vi "XNET Read (Frame Raw).vi"(0 "session in":refnum<k21>, 7 "number to read (-1)":i32=-1, 9 "timeout (0)":dbl format="%.2g", 11 "error in (no error)":errorcluster) -> (4 "session out":refnum<k21>, 6 "data":u8[](array[numeric]) format="%02x", 15 "error out":errorcluster)   [LabVIEW 2018]
doc: "Reads data from a session as an array of raw bytes. The session must use a mode of Frame Input Stream, Frame Input Queued, or Frame Input Single-Point."
uses:
  nixlvapi.dll
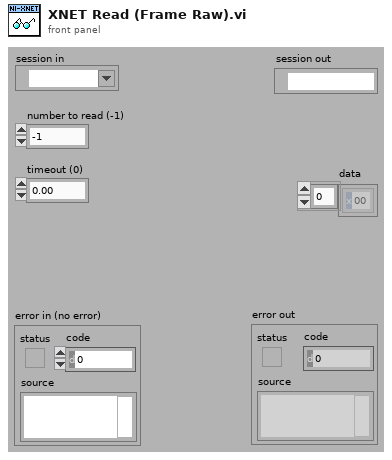
[diagram p1: front panel]
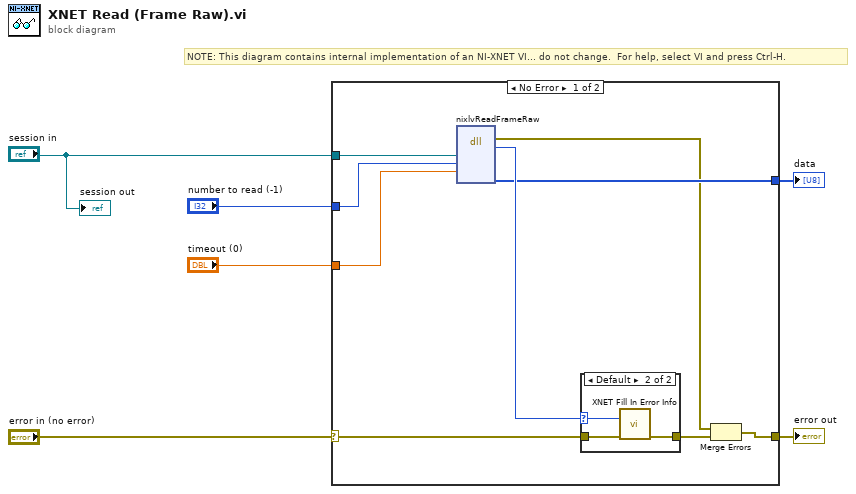
[diagram p0: block diagram]
diagram:
  # "NOTE: This diagram contains internal implementation of an NI-XNET VI... do not change.  For help, select VI and press Ctrl-H."
  n1 = case shown="No Error" "error in (no error)" {
    selector: "error in (no error)" -> [w14 w20]
    tunnel: "session in" -> [w15 _]
    tunnel: [w8 w20] -> w6
    tunnel: "number to read (-1)" -> [w11 _]
    tunnel: "timeout (0)" -> [w10 _]
    tunnel: [w9 _] -> w1
    frame No Error {
      n2 = dll-call lib="nixlvapi.*" fn="nixlvReadFrameRaw"("sessionRef"=w15, "numberToRead"=w11, "timeout"=w10) -> (error out=w7:errorcluster, "return type"=w12:i32, "lvData"=w9:u8[])  [unwired: 6 in, 2 out]
      n3 = case shown="Default" w12 {
        selector: w12 -> [_ w17]
        tunnel: w14 -> [w16 w18]
        tunnel: [w16 w19] -> w13
        frame 0 {
        }
        frame Default {
          n4 = call "XNET Fill In Error Info.vi"("status code"=w17, "error in"=w18) -> ("error out"=w19:errorcluster)  [unwired: 13 out]
        }
      }
      n5 = Merge Errors(w7, w13) -> (w8:errorcluster)
    }
    frame Error {
    }
  }
  "error out" <- w6
  "data" <- w1
  "session out" <- "session in"
